vi "QueueMidi3.vi"() -> ()   [LabVIEW 2014]
uses:
  Controls/MidiCommand.ctl
panel:
  out "Midi Command":T1={"Function"=enum."Empty", "Channel"=0, "Data Byte 1"=170, "Data Byte 2"=170}
  in  "Queue Name":string="Midi In"
  in  "error in (no error)":errorcluster
  in  "stop":bool
  out "Timeouts Occured":i32
  out "Messages Queued":i32
  in  "Character Count":u32=1
  in  "Timeout (ms)\n(-1: None)":i32=1000
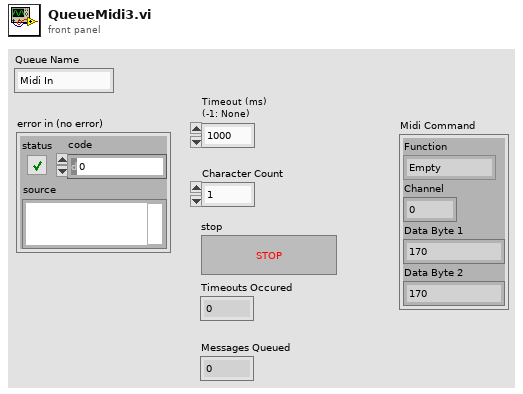
[diagram p1: front panel]
types:
  T1 = typedef "MidiCommand.ctl" = cluster{"Function":enum16{"Empty", "Note Off", "Note On", "Polyphonic Aftertouch", "Control/Mode Change", "Program Change", "Channel Aftertouch", "Pitch Bend Change", "System"}, "Channel":u8, "Data Byte 1":u8, "Data Byte 2":u8}
  T2 = cluster{"Invert Polarity?":bool, "baud rate (9600)":u32, "data bits (8)":u16, "parity (0:none)":u16, "stop bits (10: 1 bit)":u16}
  T3 = enum16{"Empty", "Note Off", "Note On", "Polyphonic Aftertouch", "Control/Mode Change", "Program Change", "Channel Aftertouch", "Pitch Bend Change", "System"}
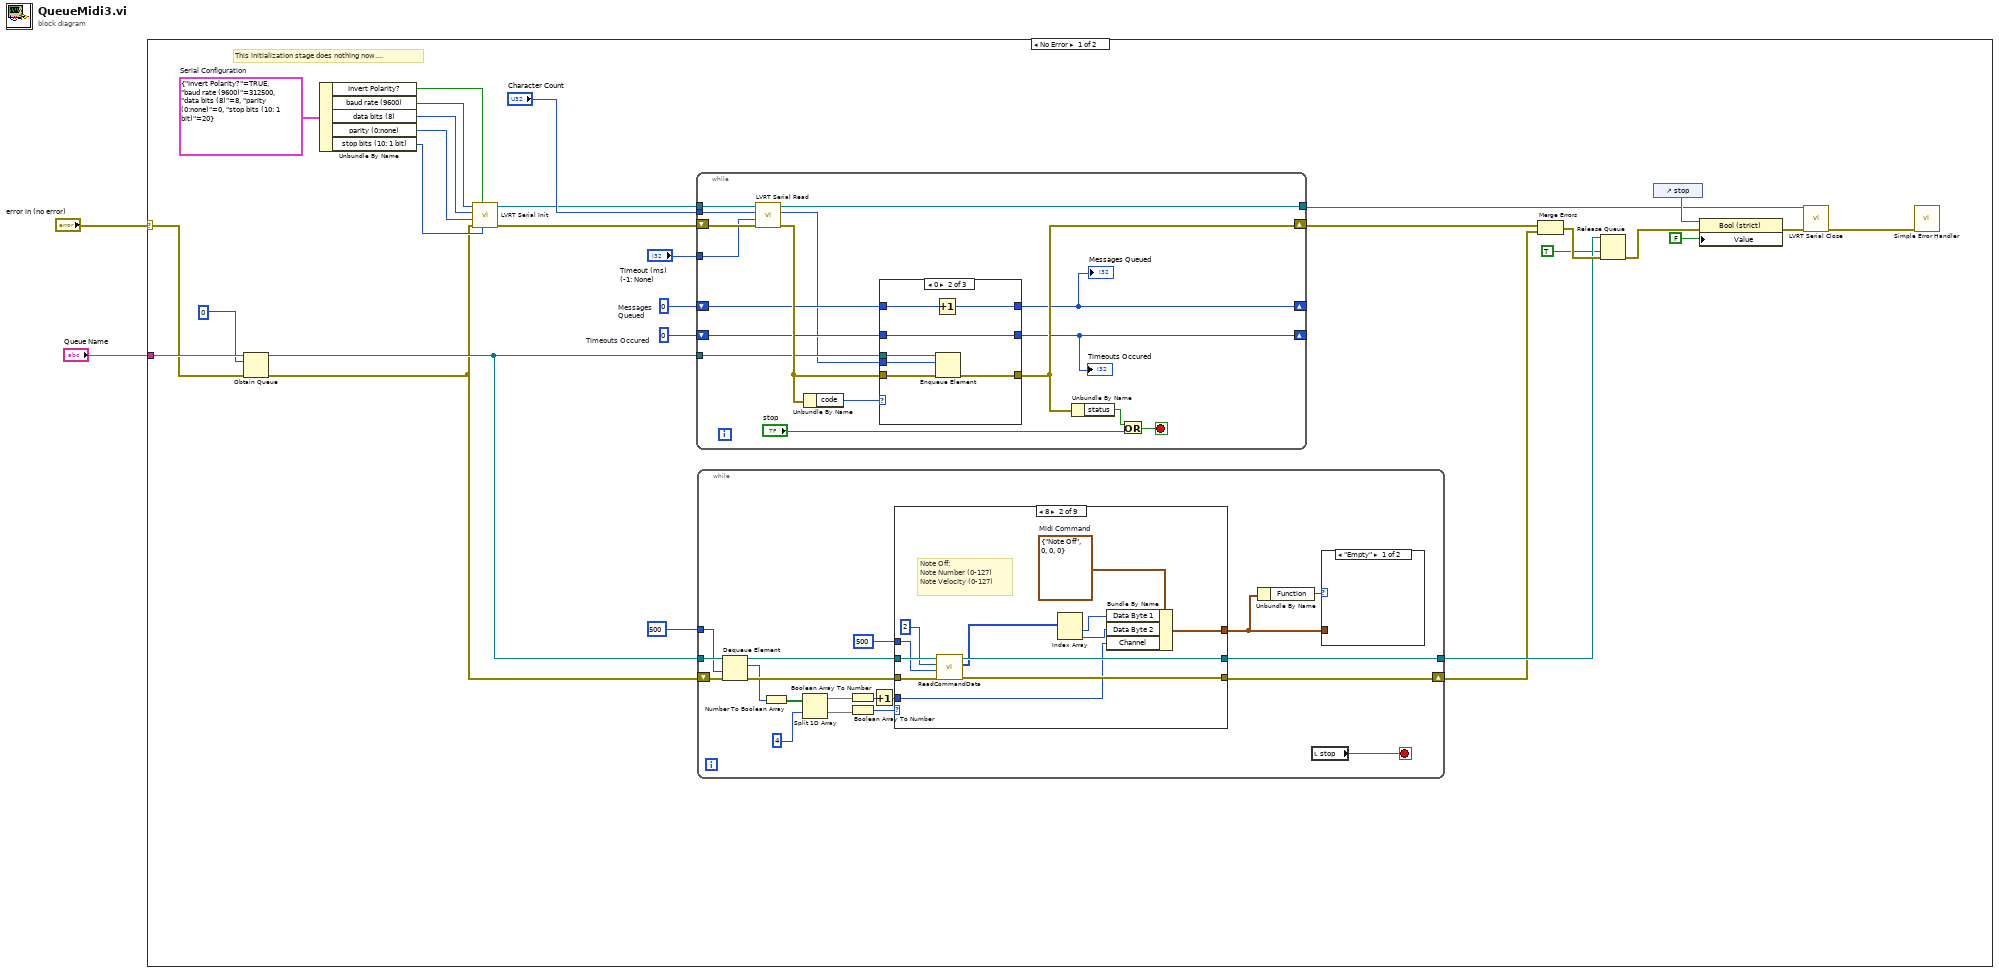
[diagram p0: block diagram]
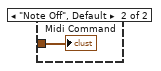
[diagram p2: hidden frame]
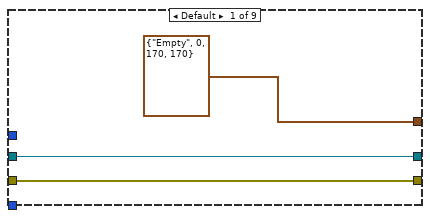
[diagram p3: hidden frame]
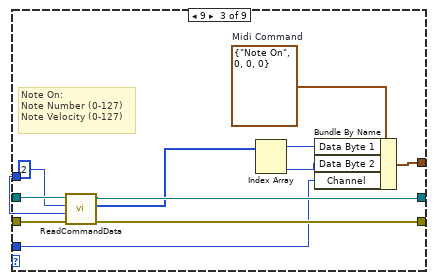
[diagram p4: hidden frame]
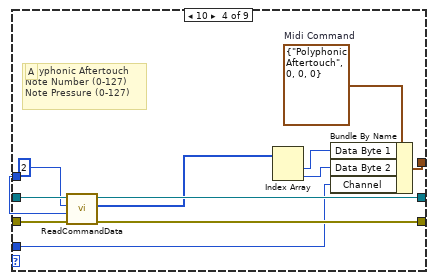
[diagram p5: hidden frame]
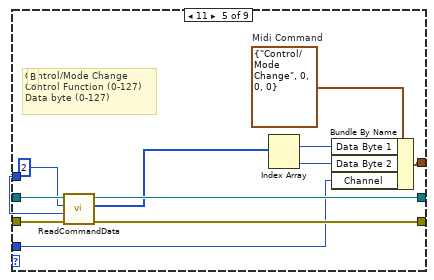
[diagram p6: hidden frame]
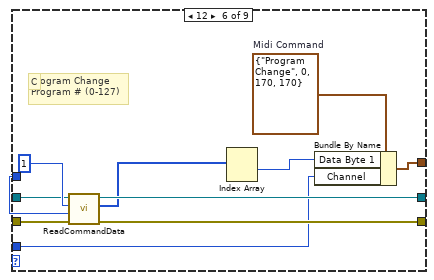
[diagram p7: hidden frame]
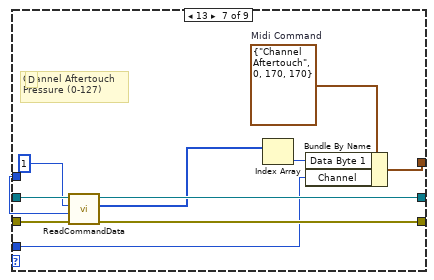
[diagram p8: hidden frame]
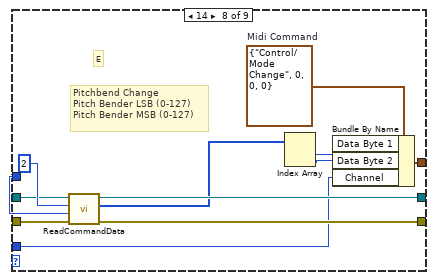
[diagram p9: hidden frame]
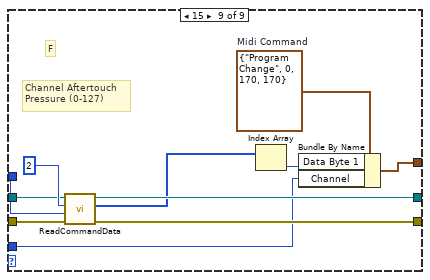
[diagram p10: hidden frame]
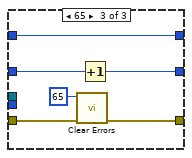
[diagram p12: hidden frame]
diagram:
  n1 = case shown="No Error" "error in (no error)" {
    selector: "error in (no error)" -> [w20 _]
    tunnel: "Queue Name" -> [w21 _]
    frame No Error {
      w18 = 0  # Messages Queued
      w19 = 0  # Timeouts Occured
      w31 = T2 {"Invert Polarity?"=TRUE, "baud rate (9600)"=312500, "data bits (8)"=8, "parity (0:none)"=0, "stop bits (10: 1 bit)"=20}  # Serial Configuration
      # "This initialization stage does nothing now...."
      n2 = Obtain Queue(name (unnamed)=w21, element data type=u8 0, error in (no error)=w20) -> (queue out=w17:refnum<queue>, error out=w16:errorcluster)  [unwired: 2 in, 1 out]
      n3 = Unbundle By Name(w31) -> ("Invert Polarity?"=w25:bool, "baud rate (9600)"=w29:u32, "data bits (8)"=w28:u16, "parity (0:none)"=w27:u16, "stop bits (10: 1 bit)"=w26:u16)
      n4 = call "LVRT Serial Init.vi"("stop bits (10: 1 bit)"=w26, "Invert Polarity?"=w25, "error in (no error)"=w16, "parity (0:none)"=w27, "data bits (8)"=w28, "baud rate (9600)"=w29) -> ("error out"=w23:errorcluster, "FPGA Main Reference Out"=w24:refnum<k20>)  [unwired: 4 in]
      n5 = while {
        shift-right: [w152] -> w13
        shift-left: w23 -> [w159]
        tunnel: "Character Count" -> [w160]
        tunnel: w24 -> [w161]
        tunnel: [w158] -> w10
        tunnel: "Timeout (ms)\n(-1: None)" -> [w157]
        tunnel: w17 -> [w154]
        shift-right: [w151] -> _
        shift-left: w19 -> [w153]
        shift-right: [w149] -> _
        shift-left: w18 -> [w150]
        stop <- w164 stop-if-true
        n6 = call "LVRT Serial Read.vi"("error in (no error)"=w159, "Timeout (ms) (-1: no timeout)"=w157, "Bytes to Read"=w160, "FPGA Main Ref"=w161) -> ("error out"=w155:errorcluster, "Read: Char"=w148:u8, "FPGA Main Ref Out"=w158:refnum<k20>)  [unwired: 5 out]
        n7 = Unbundle By Name(w155) -> ("code"=w156:i32)
        n8 = case shown="0" w156 {
          tunnel: w155 -> [w167 w173 w180]
          tunnel: w154 -> [_ w174 _]
          tunnel: [w167 w172 w179] -> w152
          tunnel: w153 -> [w166 w171 w177]
          tunnel: [w166 w171 w176] -> w151
          tunnel: w150 -> [w165 w170 w175]
          tunnel: [w165 w169 w175] -> w149
          tunnel: w148 -> [_ w168 _]
          frame 1, Default {
          }
          frame 0 {
            n9 = Increment(x=w170) -> (x+1=w169:i32)
            n10 = Enqueue Element(queue=w174, element=w168, error in (no error)=w173) -> (error out=w172:errorcluster)  [unwired: 1 in, 2 out]
          }
          frame 65 {
            n11 = call <vilib>:"Clear Errors.vi"("error in (no error)"=w180, "specific error code to clear (0: all)"=65) -> ("error out"=w179:errorcluster)  [unwired: 4 in, 1 out]
            n12 = Increment(x=w177) -> (x+1=w176:i32)
          }
        }
        "Timeouts Occured" <- w151
        "Messages Queued" <- w149
        n13 = Unbundle By Name(w152) -> ("status"=w163:bool)
        n14 = Or(x=w163, y="stop") -> (x .or. y?=w164:bool)
      }
      n15 = while {
        tunnel: w17 -> [w50]
        shift-right: [w32] -> w6
        shift-left: w16 -> [w45]
        tunnel: [w33] -> w7
        tunnel: 500 ("timeout in ms (-1)") -> [w42]
        stop <- w49 stop-if-true
        n16 = Dequeue Element(queue=w50, timeout in ms (-1)=w42, error in (no error)=w45) -> (queue out=w43:refnum<queue>, element=w36:u8, error out=w44:errorcluster)  [unwired: 1 out]
        n17 = Number To Boolean Array(number=w36) -> (Boolean array=w39:bool[])
        n18 = Split 1D Array(array=w39, index=4) -> (first subarray=w37:bool[], second subarray=w38:bool[])
        n19 = Boolean Array To Number(Boolean array=w37) -> (number=w41:u32)
        n20 = Boolean Array To Number(Boolean array=w38) -> (number=w47:u32)
        n21 = Increment(x=w41) -> (x+1=w40:u32)
        n22 = case shown="8" w47 {
          tunnel: [w53 w65 w75 w87 w100 w111 w122 w134 w146] -> w33
          tunnel: [w54 w57 w78 w89 w101 w112 w123 w135 w147] -> w32
          tunnel: w44 -> [w54 w66 w77 w90 w102 w113 w124 w136 w145]
          tunnel: w43 -> [w53 w64 w76 w88 w99 w109 w121 w132 w143]
          tunnel: 500 ("timeout in ms (-1)") -> [_ w62 w73 w85 w97 w108 w119 w131 w142]
          tunnel: [T1 {"Function"=enum."Empty", "Channel"=0, "Data Byte 1"=170, "Data Byte 2"=170} ("Midi Command") w60 w70 w83 w94 w106 w116 w128 w139] -> w34
          tunnel: w40 -> [_ w55 w67 w79 w92 w105 w114 w127 w137]
          frame Default {
          }
          frame 8 {
            w61 = T1 {"Function"=enum."Note Off", "Channel"=0, "Data Byte 1"=0, "Data Byte 2"=0}  # Midi Command
            # "Note Off: \nNote Number (0-127)\nNote Velocity (0-127)"
            n23 = call "ReadCommandData.vi"("error in (no error)"=w66, "timeout in ms (-1)"=w62, "Messages To Read"=u32 2, "Queue in"=w64) -> ("error out"=w57:errorcluster, "Data Bytes"=w56:u8[], "Queue in 2"=w65:refnum<queue>)  [unwired: 5 in]
            n24 = Index Array(array=w56) -> (element #1=w59:u8, element #2=w58:u8)  [unwired: 2 in]
            n25 = Bundle By Name(cluster=w61, "Data Byte 1"=w59, "Data Byte 2"=w58, "Channel"=w55) -> (w60:T1)
          }
          frame 9 {
            w71 = T1 {"Function"=enum."Note On", "Channel"=0, "Data Byte 1"=0, "Data Byte 2"=0}  # Midi Command
            # "Note On: \nNote Number (0-127)\nNote Velocity (0-127)"
            n26 = call "ReadCommandData.vi"("error in (no error)"=w77, "timeout in ms (-1)"=w73, "Messages To Read"=u32 2 ("byte count"), "Queue in"=w76) -> ("error out"=w78:errorcluster, "Data Bytes"=w68:u8[], "Queue in 2"=w75:refnum<queue>)  [unwired: 5 in]
            n27 = Index Array(array=w68) -> (element #1=w72:u8, element #2=w69:u8)  [unwired: 2 in]
            n28 = Bundle By Name(cluster=w71, "Data Byte 1"=w72, "Data Byte 2"=w69, "Channel"=w67) -> (w70:T1)
          }
          frame 10 {
            w84 = T1 {"Function"=enum."Polyphonic Aftertouch", "Channel"=0, "Data Byte 1"=0, "Data Byte 2"=0}  # Midi Command
            # "A"
            # "Polyphonic Aftertouch\nNote Number (0-127)\nNote Pressure (0-127)"
            n29 = call "ReadCommandData.vi"("error in (no error)"=w90, "timeout in ms (-1)"=w85, "Messages To Read"=u32 2 ("byte count"), "Queue in"=w88) -> ("error out"=w89:errorcluster, "Data Bytes"=w80:u8[], "Queue in 2"=w87:refnum<queue>)  [unwired: 5 in]
            n30 = Index Array(array=w80) -> (element #1=w82:u8, element #2=w81:u8)  [unwired: 2 in]
            n31 = Bundle By Name(cluster=w84, "Data Byte 1"=w82, "Data Byte 2"=w81, "Channel"=w79) -> (w83:T1)
          }
          frame 11 {
            w96 = T1 {"Function"=enum."Control/Mode Change", "Channel"=0, "Data Byte 1"=0, "Data Byte 2"=0}  # Midi Command
            # "B"
            # "Control/Mode Change\nControl Function (0-127)\nData byte (0-127)"
            n32 = call "ReadCommandData.vi"("error in (no error)"=w102, "timeout in ms (-1)"=w97, "Messages To Read"=u32 2 ("byte count"), "Queue in"=w99) -> ("error out"=w101:errorcluster, "Data Bytes"=w91:u8[], "Queue in 2"=w100:refnum<queue>)  [unwired: 5 in]
            n33 = Index Array(array=w91) -> (element #1=w95:u8, element #2=w93:u8)  [unwired: 2 in]
            n34 = Bundle By Name(cluster=w96, "Data Byte 1"=w95, "Data Byte 2"=w93, "Channel"=w92) -> (w94:T1)
          }
          frame 12 {
            w107 = T1 {"Function"=enum."Program Change", "Channel"=0, "Data Byte 1"=170, "Data Byte 2"=170}  # Midi Command
            # "C"
            # "Program Change\nProgram # (0-127)"
            n35 = call "ReadCommandData.vi"("error in (no error)"=w113, "timeout in ms (-1)"=w108, "Messages To Read"=u32 1 ("byte count"), "Queue in"=w109) -> ("error out"=w112:errorcluster, "Data Bytes"=w103:u8[], "Queue in 2"=w111:refnum<queue>)  [unwired: 5 in]
            n36 = Index Array(array=w103) -> (element #1=w104:u8)  [unwired: 2 in, 1 out]
            n37 = Bundle By Name(cluster=w107, "Data Byte 1"=w104, "Channel"=w105) -> (w106:T1)
          }
          frame 13 {
            w117 = T1 {"Function"=enum."Channel Aftertouch", "Channel"=0, "Data Byte 1"=170, "Data Byte 2"=170}  # Midi Command
            # "Channel Aftertouch\nPressure (0-127)"
            # "D"
            n38 = call "ReadCommandData.vi"("error in (no error)"=w124, "timeout in ms (-1)"=w119, "Messages To Read"=u32 1 ("byte count"), "Queue in"=w121) -> ("error out"=w123:errorcluster, "Data Bytes"=w115:u8[], "Queue in 2"=w122:refnum<queue>)  [unwired: 5 in]
            n39 = Index Array(array=w115) -> (element=w118:u8)  [unwired: 1 in]
            n40 = Bundle By Name(cluster=w117, "Data Byte 1"=w118, "Channel"=w114) -> (w116:T1)
          }
          frame 14 {
            w130 = T1 {"Function"=enum."Control/Mode Change", "Channel"=0, "Data Byte 1"=0, "Data Byte 2"=0}  # Midi Command
            # "E"
            # "Pitchbend Change\nPitch Bender LSB (0-127)\nPitch Bender MSB (0-127)"
            n41 = call "ReadCommandData.vi"("error in (no error)"=w136, "timeout in ms (-1)"=w131, "Messages To Read"=u32 2 ("byte count"), "Queue in"=w132) -> ("error out"=w135:errorcluster, "Data Bytes"=w125:u8[], "Queue in 2"=w134:refnum<queue>)  [unwired: 5 in]
            n42 = Index Array(array=w125) -> (element #1=w129:u8, element #2=w126:u8)  [unwired: 2 in]
            n43 = Bundle By Name(cluster=w130, "Data Byte 1"=w129, "Data Byte 2"=w126, "Channel"=w127) -> (w128:T1)
          }
          frame 15 {
            w141 = T1 {"Function"=enum."Program Change", "Channel"=0, "Data Byte 1"=170, "Data Byte 2"=170}  # Midi Command
            # "F"
            # "Channel Aftertouch\nPressure (0-127)"
            n44 = call "ReadCommandData.vi"("error in (no error)"=w145, "timeout in ms (-1)"=w142, "Messages To Read"=u32 2 ("byte count"), "Queue in"=w143) -> ("error out"=w147:errorcluster, "Data Bytes"=w138:u8[], "Queue in 2"=w146:refnum<queue>)  [unwired: 5 in]
            n45 = Index Array(array=w138) -> (element=w140:u8)  [unwired: 1 in]
            n46 = Bundle By Name(cluster=w141, "Data Byte 1"=w140, "Channel"=w137) -> (w139:T1)
          }
        }
        n47 = Unbundle By Name(w34) -> ("Function"=w35:T3)
        n48 = local read "stop"() -> (w49:bool)
        n49 = case shown="\"Empty\"" w35 {
          tunnel: w34 -> [_ w51]
          frame "Empty" {
          }
          frame "Note Off", Default {
            "Midi Command" <- w51
          }
        }
      }
      n50 = Merge Errors(w13, w6) -> (w9:errorcluster)
      n51 = Release Queue(queue=w7, force destroy? (F)=TRUE, error in (no error)=w9) -> (error out=w8:errorcluster)  [unwired: 2 out]
      n52 = control-ref of="stop"() -> (w15:refnum<vi>)
      n53 = property class="Bool (strict)"(reference=w15, error in=w8, "Value"=FALSE) -> (error out=w12:errorcluster)  [unwired: 1 out]
      n54 = call "LVRT Serial Close.vi"("error out"=w12, "FPGA Main Ref"=w10) -> ("error out"=w11:errorcluster)  [unwired: 9 in]
      n55 = call <vilib>:"Simple Error Handler.vi"("error in (no error)"=w11) -> ()  [unwired: 4 in, 5 out]
    }
    frame Error {
    }
  }
